vi "NiFpga_HdlFifo_WriteBool.vi"(6 "timeout":u32, 7 "error in (no error)":errorcluster, 8 "data in":bool[](array[boolean]), 9 "fifo number":u32, 10 "fpga vi reference in":refnum<k20>) -> (0 "error out":errorcluster, 1 "empty elements remaining":u64, 3 "fpga vi reference out":refnum<k20>)   [LabVIEW 2023]
doc: "Dynamically reads the register at the provided offset. Set check for errors to true to check for errors such as if the register offset is invalid or if the register is running in an external clock domain that might not be running."
uses:
  NiFpga.dll
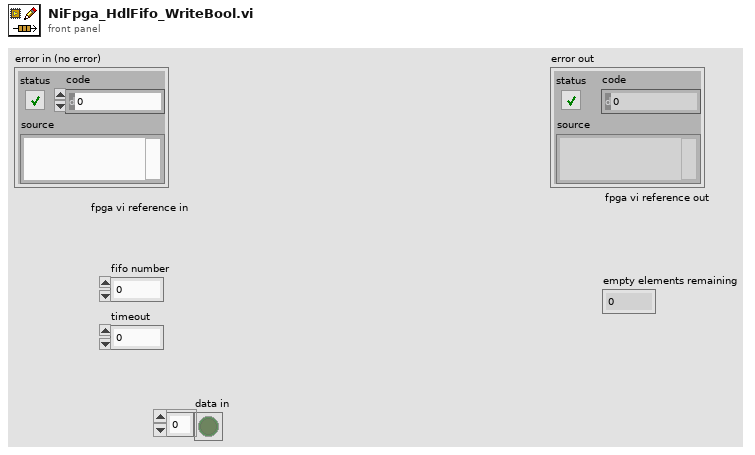
[diagram p1: front panel]
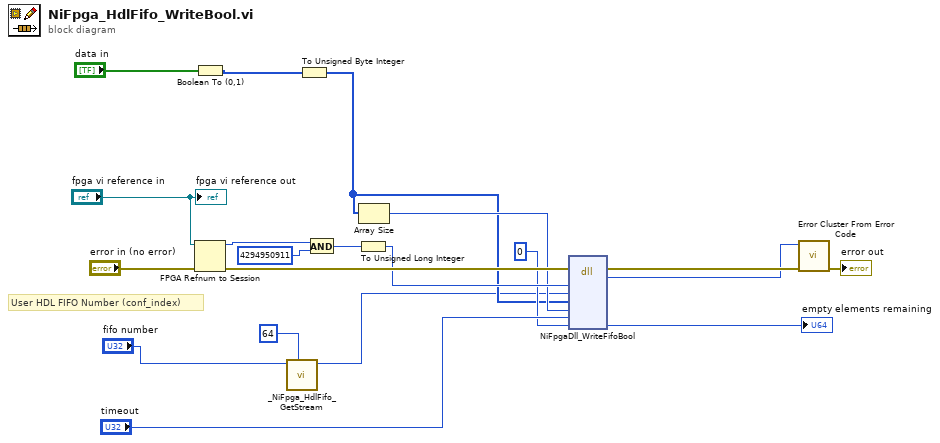
[diagram p0: block diagram]
diagram:
  # "User HDL FIFO Number (conf_index)"
  n1 = Boolean To (0,1)(Boolean="data in") -> (0, 1=w5:i16[])
  n2 = FPGA Refnum to Session(4:"error in (no error)", 7:"fpga vi reference in") -> (0:w15:errorcluster, 3:w17:u64)
  n3 = call "_NiFpga_HdlFifo_GetStream.vi"("NUM_DMA_CHANNELS"=u32 64, "Fifo Number"="fifo number") -> ("Fifo Stream"=w2:u32)  [unwired: 9 in]
  n4 = To Unsigned Byte Integer(number=w5) -> (unsigned 8bit integer=w4:u8[])
  n5 = And(x=w17, y=u64 4294950911) -> (x .and. y?=w10:u64)
  n6 = To Unsigned Long Integer(number=w10) -> (unsigned 32bit integer=w9:u32)
  n7 = Array Size(array=w4) -> (size(s)=w8:i32)
  n8 = dll-call lib="NiFpga.*" fn="NiFpgaDll_WriteFifoBool"(error in=w15, "session"=w9, "fifo"=w2, "data"=w4, "numberOfElements"=w8, "timeout"="timeout", "emptyElementsRemainining"=u64 0) -> (error out=w14:errorcluster, "return type"=w13:i32, "emptyElementsRemainining"=→"empty elements remaining":u64)  [unwired: 7 in, 1 out]
  n9 = call <vilib>:"Error Cluster From Error Code.vi"("error in (no error)"=w14, "error code (0)"=w13) -> ("error out"=→"error out":errorcluster)  [unwired: 7 in]
  "fpga vi reference out" <- "fpga vi reference in"
